vi "simple_math_operation.vi"() -> ()   [LabVIEW 2021]
panel:
  out "result":dbl
  in  "input":dbl
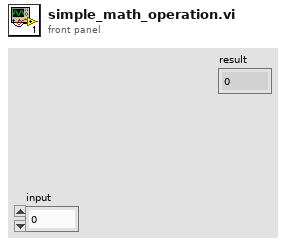
[diagram p1: front panel]
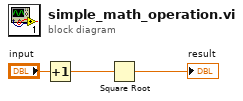
[diagram p0: block diagram]
diagram:
  n1 = Increment(x="input") -> (x+1=w2:dbl)
  n2 = Square Root(x=w2) -> (sqrt(x)=→"result":dbl)
